vi "Manual Test.vi"() -> ()   [LabVIEW 2020, in "ChromTech Series I Drivers.lvlib"]
uses:
  <instrlib>/RxnRover/ChromtechSeriesIDriver/ChromTech Series I Drivers.lvlib
panel:
  in  "Retry Attempts":i32
  out "error out":errorcluster
  in  "Stop Pump":bool
  in  "Start Pump":bool
  in  "Get User Compensation":bool
  out "Current User Compensation":dbl
  in  "stop":bool
  in  "error in (no error)":errorcluster
  in  "Fast Comms":bool
  in  "Get Current Status":bool
  out "Pressure Units":string
  out "Lower Pressure Limit":dbl
  out "Upper Pressure Limit":dbl
  in  "Get Pump Information":bool
  out "Lower Pressure Fault":bool
  out "Motor Stall":bool
  out "Keypad Enabled":bool
  out "Upper Pressure Fault":bool
  out "In Prime":bool
  out "Running":bool
  out "Head Identifier":string
  out "Pressure Compensation":i32
  out "Current Flow Rate":dbl
  out "Current Pressure":dbl
  in  "Get Current Conditions":bool
  in  "Get Firmware Details":bool
  out "Firmware Version":string
  out "Firmware Part Number":dbl
  in  "Set User Comp":bool
  in  "User Compensation":dbl=100.0
  in  "VISA resource name":refnum<visa-resource-name>
  in  "Set Flow Rate":bool
  in  "Flow Rate":dbl
  # "Teledyne SSI MX-Class Pump"
  # "Set Conditions"
  # "Current Status"
  # "Firmware Information"
  # "Still Under constuction. Should probably be reworked into state machine and \nexplicitly make a test button for each driver VI."
  # "Get Conditions"
  # "Pump Information"
  # "Pump Control"
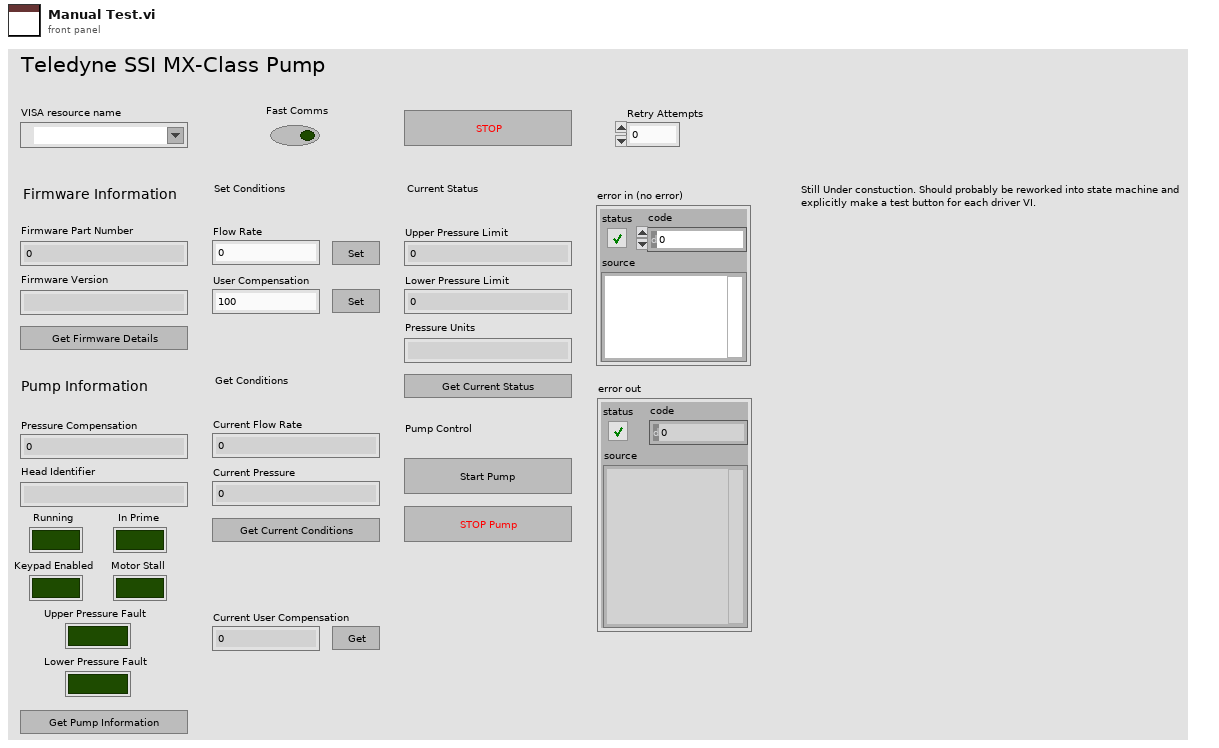
[diagram p1: front panel]
types:
  T1 = cluster{"Baud Rate":u32, "Parity":u16, "Flow Control":u16, "Data Bits":u16, "Stop Bits":u16}
  T2 = cluster{"Flow rate":dbl, "Running":bool, "Pressure Comp":i32, "Head ID":string, "Upper Pressure Fault":bool, "Lower Pressure Fault":bool, "In Prime":bool, "Keypad Enabled":bool, "Motor Stall Fault":bool, "Pump Run Input":bool, "Pump Stop Input":bool, "Control Mode":enum16{"LOCAL", "REMOTE"}}
  T3 = cluster{"Flow rate":dbl, "Upper Pressure Limit":dbl, "Lower Pressure Limit":dbl, "Pressure Units":string, "Running?":bool}
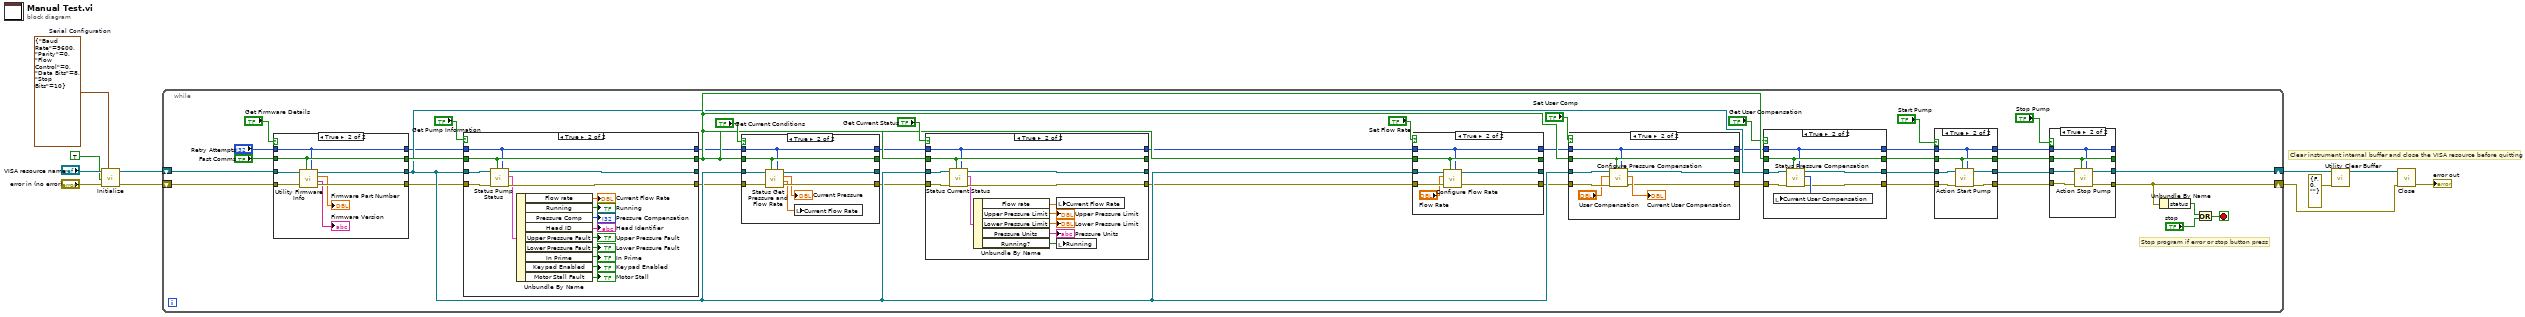
[diagram p0: block diagram]
diagram:
  w6 = T1 {"Baud Rate"=9600, "Parity"=0, "Flow Control"=0, "Data Bits"=8, "Stop Bits"=10}  # Serial Configuration
  # "Clear instrument internal buffer and close the VISA resource before quitting"
  n1 = call <instrlib>:"Initialize.vi"("Serial Configuration"=w6, "error in (no error)"="error in (no error)", "Fast Comms (F)"=TRUE, "VISA resource name"="VISA resource name") -> ("error out"=w8:errorcluster, "VISA resource name out"=w10:refnum<visa-resource-name>)  [unwired: 6 in]
  n2 = while {
    shift-right: [w21] -> w1
    shift-left: w8 -> [w51]
    shift-right: [w22] -> w3
    shift-left: w10 -> [w40]
    stop <- w25 stop-if-true
    # "Stop program if error or stop button press"
    n3 = case shown="True" "Get Firmware Details" {
      tunnel: w40 -> [w157 w165]
      tunnel: w51 -> [w156 w164]
      tunnel: [w157 w163] -> w43
      tunnel: [w156 w162] -> w39
      tunnel: [w155 w159] -> w50
      tunnel: "Fast Comms" -> [w155 w159]
      tunnel: "Retry Attempts" -> [w154 w158]
      tunnel: [w154 w158] -> w19
      frame False {
      }
      frame True {
        n4 = call <instrlib>:"Utility Firmware Info.vi"("Retry Attempts (0)"=w158, "Fast Comms (F)"=w159, "error in"=w164, "VISA resource name"=w165) -> ("error out"=w162:errorcluster, "Firmware Version"=→"Firmware Version":string, "Firmware Part Number"=→"Firmware Part Number":dbl, "VISA resource name out"=w163:refnum<visa-resource-name>)  [unwired: 4 in]
      }
    }
    n5 = case shown="True" "Get Pump Information" {
      tunnel: w43 -> [w138 w153]
      tunnel: [w138 w152] -> _
      tunnel: w39 -> [w137 w151]
      tunnel: [w137 w151] -> w38
      tunnel: w50 -> [w136 w140]
      tunnel: [w136 w140] -> w44
      tunnel: w19 -> [w135 w139]
      tunnel: [w135 w139] -> w18
      frame False {
      }
      frame True {
        n6 = call <instrlib>:"Status Pump Status.vi"("Retry Attempts (0)"=w139, "Fast Comms (F)"=w140, "error in (no error)"=w151, "VISA resource name"=w153) -> ("Status Cluster"=w150:T2, "VISA resource name out"=w152:refnum<visa-resource-name>)  [unwired: 5 in, 1 out]
        n7 = Unbundle By Name(w150) -> ("Flow rate"=→"Current Flow Rate":dbl, "Running"=→"Running":bool, "Pressure Comp"=→"Pressure Compensation":i32, "Head ID"=→"Head Identifier":string, "Upper Pressure Fault"=→"Upper Pressure Fault":bool, "Lower Pressure Fault"=→"Lower Pressure Fault":bool, "In Prime"=→"In Prime":bool, "Keypad Enabled"=→"Keypad Enabled":bool, "Motor Stall Fault"=→"Motor Stall":bool)
      }
    }
    n8 = case shown="True" "Get Current Conditions" {
      tunnel: w43 -> [w125 w134]
      tunnel: [w125 w133] -> _
      tunnel: w38 -> [w124 w132]
      tunnel: [w124 w131] -> w37
      tunnel: w44 -> [w126 w128]
      tunnel: [w126 w128] -> _
      tunnel: w18 -> [w123 w127]
      tunnel: [w123 w127] -> w17
      frame False {
      }
      frame True {
        n9 = call <instrlib>:"Status Get Pressure and Flow Rate.vi"("Retry Attempts (0)"=w127, "Fast Comms (F)"=w128, "error in"=w132, "VISA resource name"=w134) -> ("error out"=w131:errorcluster, "Flow Rate"=w129:dbl, "Pressure"=→"Current Pressure":dbl, "VISA resource name out"=w133:refnum<visa-resource-name>)  [unwired: 4 in]
        n10 = local write "Current Flow Rate"(w129) -> ()
      }
    }
    n11 = case shown="True" "Get Current Status" {
      tunnel: w44 -> [w108 w112]
      tunnel: [w108 w112] -> _
      tunnel: w43 -> [w109 w122]
      tunnel: [w109 w121] -> _
      tunnel: w37 -> [w110 w120]
      tunnel: [w110 w119] -> w36
      tunnel: w17 -> [w107 w111]
      tunnel: [w107 w111] -> w16
      frame False {
      }
      frame True {
        n12 = call <instrlib>:"Status Current Status.vi"("Retry Attempts (0)"=w111, "Fast Comms (F)"=w112, "error in (no error)"=w120, "VISA resource name"=w122) -> ("error out"=w119:errorcluster, "Status Cluster"=w118:T3, "VISA resource name out"=w121:refnum<visa-resource-name>)  [unwired: 5 in]
        n13 = Unbundle By Name(w118) -> ("Flow rate"=w117:dbl, "Upper Pressure Limit"=→"Upper Pressure Limit":dbl, "Lower Pressure Limit"=→"Lower Pressure Limit":dbl, "Pressure Units"=→"Pressure Units":string, "Running?"=w113:bool)
        n14 = local write "Current Flow Rate"(w117) -> ()
        n15 = local write "Running"(w113) -> ()
      }
    }
    n16 = case shown="True" "Set Flow Rate" {
      tunnel: w44 -> [w99 w101]
      tunnel: w43 -> [w98 w106]
      tunnel: w36 -> [w97 w104]
      tunnel: [w99 w101] -> _
      tunnel: [w98 w105] -> _
      tunnel: [w97 w103] -> w35
      tunnel: w16 -> [w96 w100]
      tunnel: [w96 w100] -> w15
      frame False {
      }
      frame True {
        n17 = call <instrlib>:"Configure Flow Rate.vi"("Retry Attempts (0)"=w100, "Fast Comms (F)"=w101, "error in"=w104, "Flow Input (ml/min)"="Flow Rate", "VISA resource name"=w106) -> ("error out"=w103:errorcluster, "VISA resource name out"=w105:refnum<visa-resource-name>)  [unwired: 5 in]
      }
    }
    n18 = case shown="True" "Set User Comp" {
      tunnel: w44 -> [w87 w89]
      tunnel: w43 -> [w86 w95]
      tunnel: w35 -> [w85 w93]
      tunnel: [w87 w89] -> _
      tunnel: [w86 w94] -> _
      tunnel: [w85 w90] -> w34
      tunnel: w15 -> [w84 w88]
      tunnel: [w84 w88] -> w14
      frame False {
      }
      frame True {
        n19 = call <instrlib>:"Configure Pressure Compensation.vi"("Retry Attempts (0)"=w88, "Fast Comms (F)"=w89, "error in"=w93, "Operating Pressure (PSI)"="User Compensation", "VISA resource name"=w95) -> ("error out"=w90:errorcluster, "Response Compensation"=→"Current User Compensation":dbl, "VISA resource name out"=w94:refnum<visa-resource-name>)  [unwired: 4 in]
      }
    }
    n20 = case shown="True" "Get User Compensation" {
      tunnel: w44 -> [w76 w78]
      tunnel: w43 -> [w75 w83]
      tunnel: w34 -> [w74 w81]
      tunnel: [w74 w79] -> w31
      tunnel: [w75 w82] -> w32
      tunnel: [w76 w78] -> w27
      tunnel: w14 -> [w73 w77]
      tunnel: [w73 w77] -> w13
      frame False {
      }
      frame True {
        n21 = call <instrlib>:"Status Pressure Compensation.vi"("Retry Attempts (0)"=w77, "Fast Comms (F)"=w78, "error in"=w81, "VISA resource name"=w83) -> ("error out"=w79:errorcluster, "Pressure Compensation (PSI)"=w80:i32, "VISA resource name out"=w82:refnum<visa-resource-name>)  [unwired: 5 in]
        n22 = local write "Current User Compensation"(w80) -> ()
      }
    }
    n23 = case shown="True" "Start Pump" {
      tunnel: [w66 w70] -> w29
      tunnel: w32 -> [w66 w71]
      tunnel: [w65 w69] -> w28
      tunnel: w31 -> [w65 w72]
      tunnel: [w64 w68] -> w26
      tunnel: w27 -> [w64 w68]
      tunnel: w13 -> [w63 w67]
      tunnel: [w63 w67] -> w12
      frame False {
      }
      frame True {
        n24 = call <instrlib>:"Action Start Pump.vi"("Retry Attempts (0)"=w67, "Fast Comms (F)"=w68, "error in"=w72, "VISA resource name"=w71) -> ("error out"=w69:errorcluster, "VISA resource name out"=w70:refnum<visa-resource-name>)  [unwired: 6 in]
      }
    }
    n25 = case shown="True" "Stop Pump" {
      tunnel: [w56 w60] -> w22
      tunnel: w29 -> [w56 w61]
      tunnel: [w55 w59] -> w21
      tunnel: w28 -> [w55 w62]
      tunnel: w26 -> [w54 w58]
      tunnel: [w54 w58] -> _
      tunnel: w12 -> [w53 w57]
      tunnel: [w53 w57] -> _
      frame False {
      }
      frame True {
        n26 = call <instrlib>:"Action Stop Pump.vi"("Retry Attempts (0)"=w57, "Fast Comms (F)"=w58, "error in"=w62, "VISA resource name"=w61) -> ("error out"=w59:errorcluster, "VISA resource name out"=w60:refnum<visa-resource-name>)  [unwired: 6 in]
      }
    }
    n27 = Unbundle By Name(w21) -> ("status"=w24:bool)
    n28 = Or(x=w24, y="stop") -> (x .or. y?=w25:bool)
  }
  n29 = call <instrlib>:"Utility Clear Buffer.vi"("error in (no error)"=errorcluster {"status"=FALSE, "code"=0, "source"=""}, "VISA resource name"=w3) -> ("VISA resource name out"=w5:refnum<visa-resource-name>)  [unwired: 8 in, 1 out]
  n30 = call <instrlib>:"Close.vi"("error in (no error)"=w1, "VISA resource name"=w5) -> ("error out"=→"error out":errorcluster)  [unwired: 9 in]
